vi "16.Camera.vi"() -> ()   [LabVIEW 2017]
uses:
  <vilib>/userdefined/High Color/IMAQdx.ctl
  <vilib>/vision/driver/NI_Vision_Acquisition_Software.lvlib
panel:
  out "Image":T1(plugin-control)
  in  "停止":bool
  out "Buffer Number":u32
  in  "Camera Name":T2
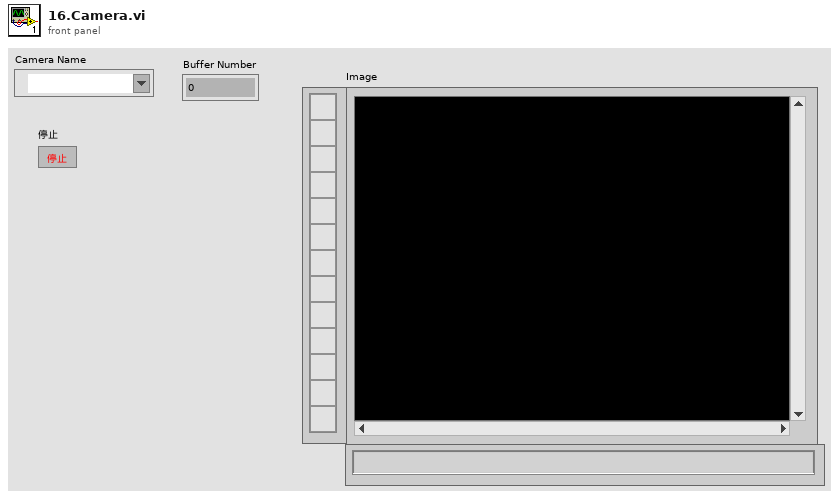
[diagram p1: front panel]
types:
  T1 = typedef "IMAQ Image.ctl" = refnum<image>
  T2 = typedef "IMAQdx.ctl" = refnum<k21>
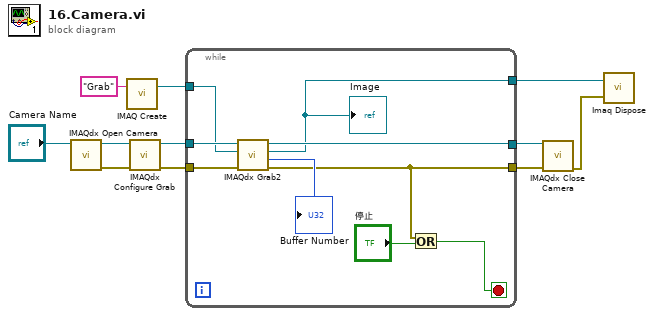
[diagram p0: block diagram]
diagram:
  n1 = call <vilib>:"IMAQdx Open Camera.vi"("Session In"="Camera Name") -> ("error out"=w11:errorcluster, "Session Out"=w10:T2)  [unwired: 9 in]
  n2 = call "IMAQ Create"("Image Name"="Grab") -> ("New Image"=w7:T1)  [unwired: 4 in, 1 out]
  n3 = call <vilib>:"IMAQdx Configure Grab.vi"("error in"=w11, "Session In"=w10) -> ("error out"=w4:errorcluster, "Session Out"=w8:T2)  [unwired: 8 in]
  n4 = while {
    tunnel: w8 -> [w20]
    tunnel: w7 -> [w19]
    tunnel: [w12] -> w5
    tunnel: w4 -> [w17]
    tunnel: [w16] -> w3
    tunnel: [w14] -> w2
    stop <- w13 stop-if-true
    n5 = call <vilib>:"IMAQdx Grab2.vi"("error in"=w17, "Image In"=w19, "Session In"=w20) -> ("error out"=w14:errorcluster, "Buffer Number Out"=→"Buffer Number":u32, "Image Out"=w12:T1, "Session Out"=w16:T2)  [unwired: 5 in]
    "Image" <- w12
    n6 = Or(x=w14, y="停止") -> (x .or. y?=w13:bool)
  }
  n7 = call <vilib>:"IMAQdx Close Camera.vi"("error in"=w2, "Session In"=w3) -> ("error out"=w1:errorcluster)  [unwired: 9 in]
  n8 = call "Imaq Dispose"("Image"=w5, "error in (no error)"=w1) -> ()  [unwired: 4 in, 1 out]
